vi "One Ball.vi"() -> ()   [LabVIEW 2014]
uses:
  Team Code/Robot Global Data.vi
panel:
  out "Angle":dbl
  out "Distance (in)":dbl
  in  "Min. Power":dbl=0.1 format="%#_13g"
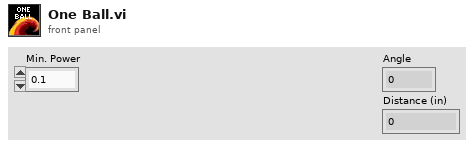
[diagram p1: front panel]
types:
  T1 = cluster{"FIRE!!!":bool, "Loader":bool, "Lock":bool, "Load":bool, "Pass":bool, "Grab":bool, "PANIC":bool, "Don't Cock":bool, "Roller Speed":dbl}
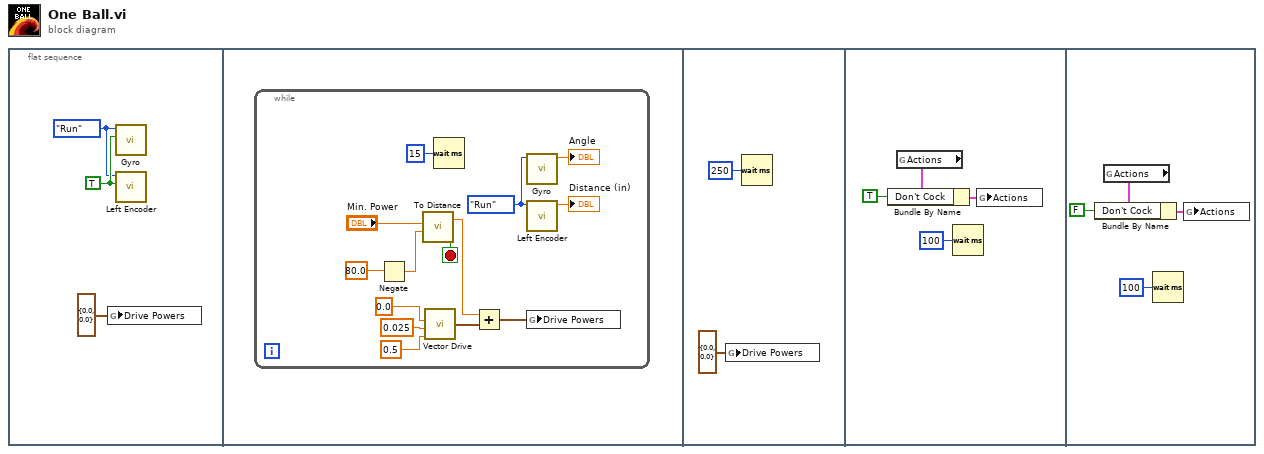
[diagram p0: block diagram]
diagram:
  n1 = flat-sequence {
    frame #0 {
      w2 = enum16{"Start", "Run", "End"}."Run" ("Enum")
      w3 = TRUE ("Reset")
      n2 = global write "Robot Global Data.vi" "Drive Powers"(cluster{"Right":dbl, "Left":dbl} {"Right"=0.0, "Left"=0.0} ("Drive Powers")) -> ()
      n3 = call "Gyro.vi"("Reset"=w3, "Enum"=w2) -> ()  [unwired: 9 in, 1 out]
      n4 = call "Left Encoder.vi"("Reset"=w3, "Enum"=w2) -> ()  [unwired: 8 in, 2 out]
    }
    frame #1 {
      n5 = while {
        stop <- w16 stop-if-true
        w9 = enum16{"Start", "Run", "End"}."Run" ("Enum")
        n6 = Negate(x=80.0) -> (-x=w7:dbl)
        n7 = call "To Distance.vi"("Destination Dist (in)"=w7, "Min. Power"="Min. Power") -> ("Reached Distance"=w16:bool, "Base Speed"=w6:dbl)  [unwired: 2 in]
        n8 = call "Vector Drive.vi"("Tolerance"=0.5, "Min. Power"=0.025, "Angle"=0.0) -> ("Motor Powers"=w12:cluster{"RMotor":dbl, "LMotor":dbl})  [unwired: 1 in]
        n9 = Wait (ms)(milliseconds to wait=u32 15) -> ()  [unwired: 1 out]
        n10 = Add(x=w6, y=w12) -> (x+y=w11:cluster{"RMotor":dbl, "LMotor":dbl})
        n11 = call "Gyro.vi"("Enum"=w9) -> ("Angle"=→"Angle":dbl)  [unwired: 10 in]
        n12 = call "Left Encoder.vi"("Enum"=w9) -> ("Distance (in)"=→"Distance (in)":dbl)  [unwired: 9 in, 1 out]
        n13 = global write "Robot Global Data.vi" "Drive Powers"(w11) -> ()
      }
    }
    frame #2 {
      n14 = global write "Robot Global Data.vi" "Drive Powers"(cluster{"Right":dbl, "Left":dbl} {"Right"=0.0, "Left"=0.0} ("Drive Powers")) -> ()
      n15 = Wait (ms)(milliseconds to wait=u32 250) -> ()  [unwired: 1 out]
    }
    frame #3 {
      n16 = global read "Robot Global Data.vi" "Actions"() -> (w22:T1)
      n17 = Bundle By Name(cluster=w22, "Don't Cock"=TRUE ("Primary Action")) -> (w23:T1)
      n18 = Wait (ms)(milliseconds to wait=u32 100) -> ()  [unwired: 1 out]
      n19 = global write "Robot Global Data.vi" "Actions"(w23) -> ()
    }
    frame #4 {
      n20 = global read "Robot Global Data.vi" "Actions"() -> (w26:T1)
      n21 = Bundle By Name(cluster=w26, "Don't Cock"=FALSE ("Primary Action")) -> (w25:T1)
      n22 = Wait (ms)(milliseconds to wait=u32 100) -> ()  [unwired: 1 out]
      n23 = global write "Robot Global Data.vi" "Actions"(w25) -> ()
    }
  }
